vi "Robot Global Data.vi"() -> ()   [LabVIEW 2019]
doc: "This global VI can contain as many global variables as you need. To create a global variable, place a control on the panel, give it a good name. To read or write to it from a VI, drag the icon to the diagram of that VI. You can also drag from the project. Click on the node to change which global you access. You shouldn't have multiple locations writing to a global or it will cause a race-condition."
uses:
  <vilib>/Rock Robotics/WPI/Camera/WPI_CameraImageSize.ctl
  <vilib>/Rock Robotics/WPI/DriverStation/WPI_DriverStationRobotMode2.ctl
  Support Code/Controls/ADIS 16448 HW Configuration.ctl
  <vilib>/Rock Robotics/WPI/SPI/WPI_SPIMode.ctl
  <vilib>/Rock Robotics/SystemInterfaces/DIO/FPGA_DIOChannel.ctl
  <vilib>/Rock Robotics/SystemInterfaces/spilib/spi_bus.ctl
panel:
  in  "Ultrasonic Scaling factor":dbl=0.000147
  in  "Speed Rate at 2 inches":dbl
  in  "Speed Rate at 6 inches":dbl
  out "Proximity Distance":dbl
  out "Data Logger":bool
  in  "Pivot Right R":dbl=0.4
  in  "Pivot Right L":dbl=0.3
  in  "Path":string
  in  "Control Panel Color Duration":dbl=4.0
  in  "Control Panel Color Set Point":dbl=0.3
  in  "Pivot Left R":dbl=0.4
  in  "Pivot Left L":dbl=0.3
  out "Correct Color":bool
  in  "Desired Color":string
  out "Color":u32(colorbox)
  out "Measured Color Name":string="Blue"
  out "Match Confidence":dbl=-inf
  out "Measured Color":cluster{"R":dbl, "G":dbl, "B":dbl}
  out "Proximity":u16(graph)
  in  "Control Panel Duration":dbl=5.5
  in  "Control Panel Set Point":dbl=0.6
  in  "ADIS16448 Data":T1={"XAngle"=-0.2168852887790008, "YAngle"=-0.11604830219780984, "ZAngle"=0.4491568601713474}
  in  "Calibration Time (sec)":u32=4
  in  "ADIS16448 HW Configuration":T2={"SPI Clock Rate (Hz)"=1000000.0, "IMU SPI Mode (3)"=enum."Mode 3 (Clk Idle High,Sample on Trailing)", "IMU Reset Pin"=enum."DIO MXP 8", "IMU SPI Bus"=enum."SPI MXP", "IMU Data Ready Pin"=enum."DIO MXP 0", "Stall Config"={"Pow2BytesPerRead"=255, "StallTicks"=1000, "CsToSclkTicks"=5}, "IMU Status LED Pin"=enum."DIO MXP 9"}
  in  "Transfer Duration":dbl=0.5
  in  "Transfer Set Point":dbl=0.6
  in  "Shooter Duration":dbl=0.5
  in  "Shooter Set Point":dbl=1.0
  in  "Intake Duration":dbl=0.5
  in  "Intake Set Point":dbl=1.0
  in  "AimDeadband":dbl=0.1 min=0.0 max=10.0 step=0.25
  in  "SteeringK":dbl(slide)=0.025362318840579712 min=0.0 max=0.25 step=0.01 scale=0.0..0.25
  in  "MinSteerCommand":dbl(slide)=0.2717391304347826 min=0.0 max=0.5 step=0.05 scale=0.0..0.5
  in  "Limelight Goal Area":dbl(slide)=1.91 min=0.1 max=2.5 step=0.25 scale=0.0..2.5
  in  "DriveK":dbl(slide)=0.5 min=0.0 max=1.0 step=0.05 scale=0.0..1.0
  in  "MaxDrive":dbl(slide)=1.0 min=0.0 max=1.0 step=0.01 scale=0.0..1.0
  in  "DriveScale":dbl(slide)=0.7556179775280899 min=0.25 max=1.0 step=0.1 scale=0.25..1.0
  in  "Steering Scale":dbl(slide)=0.6418539325842696 min=0.25 max=1.0 step=0.1 scale=0.25..1.0
  in  "MaxSpeedSlow":dbl=0.6
  in  "SlowRate":dbl=1.0
  in  "MaxTurnSlow":dbl=0.55
  in  "MaxTurnRateSlow":dbl=20.0
  in  "SlowModeSettings":i32=2
  in  "Cheezy Drive Mode":u32=2
  out "tv - valid target":dbl=1.0
  out "Op. Right Trigger 7":bool
  out "Op. Left Trigger 6":bool
  out "Op. Right Button 5":bool
  out "Op. Left Button 4":bool
  out "Op. Square 3":bool
  out "Op. X 2":bool
  out "Op. Circle 1":bool
  out "Op Triangle 0":bool
  in  "y axis Climb":dbl
  in  "x axis":dbl=-0.0
  out "D Right Triger  7":bool
  out "D Left Triger 6":bool
  out "D Right Button 5":bool
  out "D Left Button 4":bool
  out "D Square 3":bool
  out "D X 2":bool
  out "D Circle 1":bool
  out "D Triangle 0":bool
  out "tx - offsetAngle H":dbl=0.16126251220703125
  out "ty - offsetAngle V":dbl=-1.5031967163085938
  out "ta - area":dbl=1.791585087776184
  out "ts - skew":dbl=-85.46223449707031
  in  "Right Pivot":bool
  in  "Left Pivot":bool
  in  "SlowMode":u32=2
  in  "Quickturn":bool
  in  "Select Mode":dbl
  in  "Speed":dbl
  in  "Turn":dbl=-0.0
  in  "Robot Mode":T6=enum."Finish"
  in  "image size":T7=enum."320x240"
  in  "Enable Vision":bool=TRUE
  # "Cheezy Drive Settings"
  # "Drive Settings"
  # "Limelight Variables"
  # "Limelight Drive Variables"
  # "Driver Joystick Variables"
  # "Operator Joystick Variables"
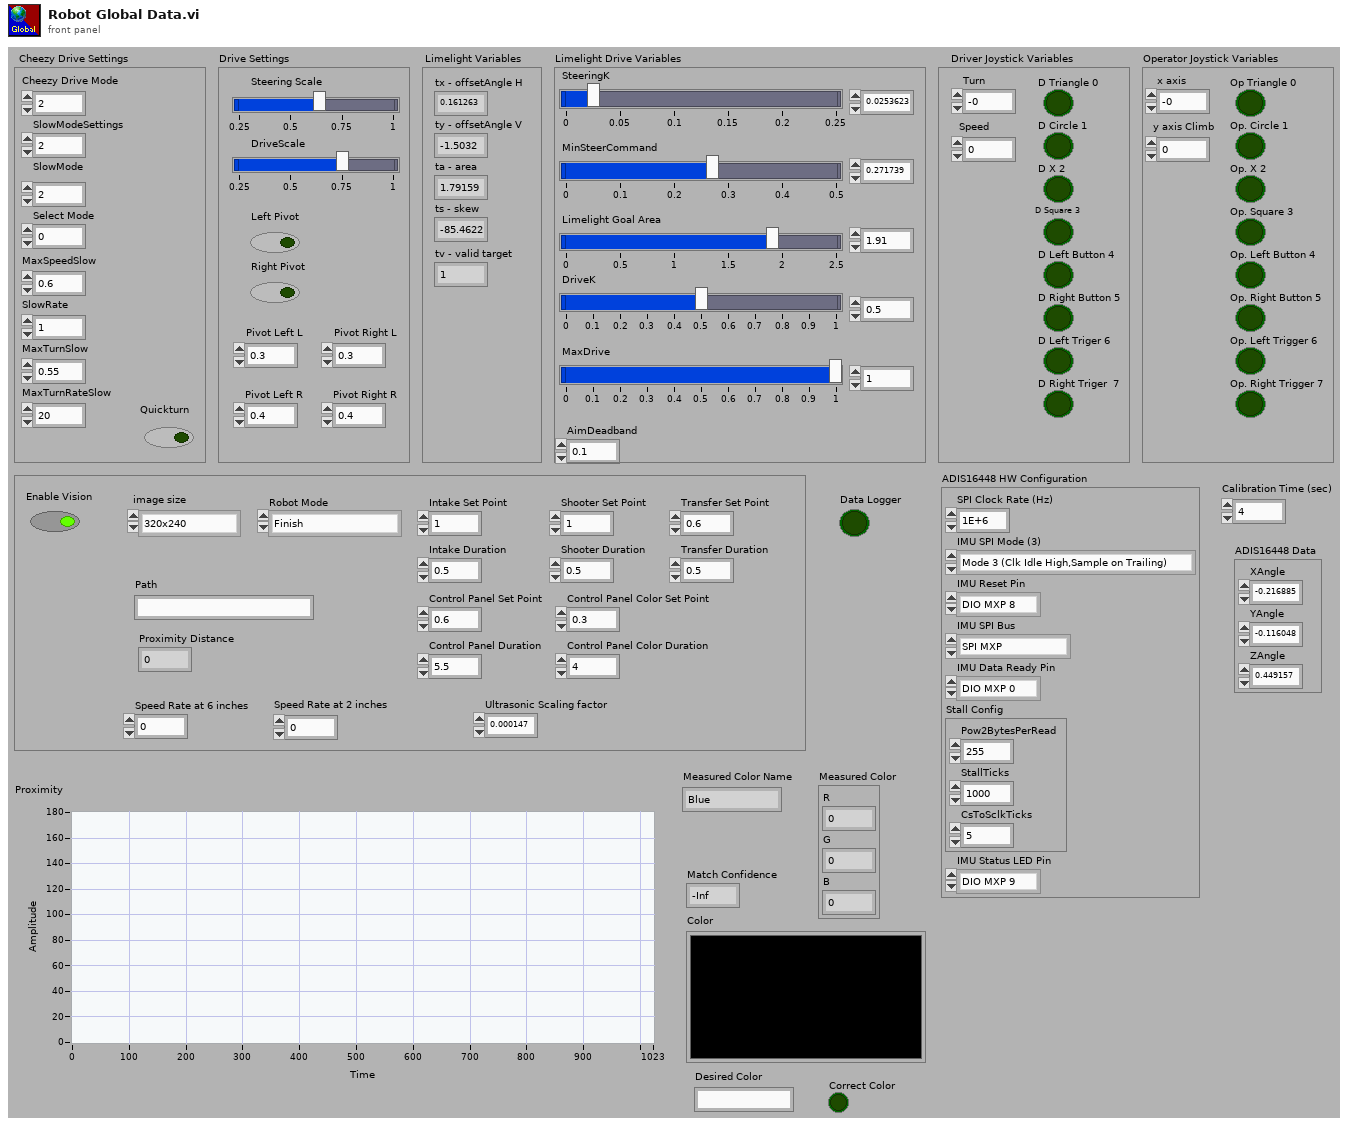
[diagram p1: front panel]
types:
  T1 = cluster{"XAngle":dbl, "YAngle":dbl, "ZAngle":dbl}
  T2 = typedef "ADIS 16448 HW Configuration.ctl" = cluster{"SPI Clock Rate (Hz)":dbl, "IMU SPI Mode (3)":T3, "IMU Reset Pin":T4, "IMU SPI Bus":T5, "IMU Data Ready Pin":T4, "Stall Config":cluster{"Pow2BytesPerRead":u8, "StallTicks":u16, "CsToSclkTicks":u8}, "IMU Status LED Pin":T4}
  T3 = typedef "WPI_SPIMode.ctl" = enum16{"Mode 0 (Clk Idle Low,Sample on Leading)", "Mode 1 (Clk Idle Low,Sample on Trailing)", "Mode 2 (Clk Idle High,Sample on Leading)", "Mode 3 (Clk Idle High,Sample on Trailing)"}
  T4 = typedef "FPGA_DIOChannel.ctl" = enum8{"DIO 0", "DIO 1", "DIO 2", "DIO 3", "DIO 4", "DIO 5", "DIO 6", "DIO 7", "DIO 8", "DIO 9", "DIO MXP 0", "DIO MXP 1", "DIO MXP 2", "DIO MXP 3", "DIO MXP 4", "DIO MXP 5", "DIO MXP 6", "DIO MXP 7", "DIO MXP 8", "DIO MXP 9", "DIO MXP 10", "DIO MXP 11", "DIO MXP 12", "DIO MXP 13", "DIO MXP 14", "DIO MXP 15", "SPI Port CS1", "SPI Port CS2", "SPI Port CS3", "SPI Port MISO", "SPI Port MOSI", "Invalid"}
  T5 = typedef "spi_bus.ctl" = enum16{"SPI On-Board, CS0", "SPI On-Board, CS1", "SPI On-Board, CS2", "SPI On-Board, CS3", "SPI MXP", "Invalid"}
  T6 = typedef "WPI_DriverStationRobotMode2.ctl" = enum16{"Autonomous Disabled", "Autonomous Enabled", "Teleop Disabled", "Teleop Enabled", "Disconnected", "Finish", "Test Disabled", "Test Enabled", "Emergency Stopped"}
  T7 = typedef "WPI_CameraImageSize.ctl" = enum16{"640x480", "320x240", "160x120", "Custom"}
diagram:
